vi "Clear message loop data.vi"(8 "error in (no error)":errorcluster, 11 "WAMP Client in":refnum<class "WAMP Client.lvclass">) -> (0 "error out":errorcluster, 3 "WAMP Clientout":refnum<class "WAMP Client.lvclass">)   [LabVIEW 2020, in "wamplv.lvlib" / "WAMP Client.lvclass"]
uses:
  WAMP Client.lvclass
  WAMP Client.lvclass/WAMP Client.ctl
  40994654-522d-4563-af25-94940d777c61.vi
  0b795402-a15f-4e31-95f5-2584284148d9.vi
  89e3171d-1602-4a33-a612-a198901d9ad6.vi
  a81c471f-8b4b-4529-bc43-673d3f160381.vi
  eb7fa446-2140-4dae-9b01-4fc8c6eccd10.vi
  40199801-e6b2-4318-9092-4349dd282dd3.vi
  6c0fe5e2-9903-440e-930a-5a8fedeab614.vi
  Private/Requests/ICallRequest/ICallRequest.lvclass
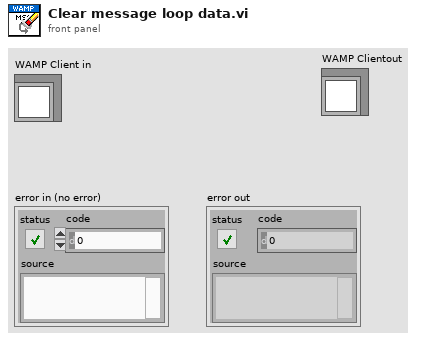
[diagram p1: front panel]
types:
  T1 = typedef "wamplv.lvlib/WAMP Client.lvclass/Message Loop Data.ctl" = cluster{"Last Request ID":u64, "Register Requests":map{u64, T2}, "Publish Requests":T3, "Endpoints Map":map{u64, T5}, "Call Requests":T6, "Subscription Requests":T7, "Subscriptions":T9, "Unsubscribe Requests":T11, "Random Request IDs":u64[], "Unregister requests map":T13}
  T2 = typedef "wamplv.lvlib/WAMP Client.lvclass/REGISTER Request Data.ctl" = cluster{"Procedure URI":string, "Options":string, "REGISTER result notifier":refnum<notifier>}
  T3 = typedef "wamplv.lvlib/WAMP Client.lvclass/Publish Requests Map.ctl" = map{u64, T4}
  T4 = typedef "wamplv.lvlib/WAMP Client.lvclass/PUBLISH Request Data.ctl" = cluster{"Topic URI":string, "Arguments":string, "ArgumentsKw":string, "Request Acknowledgement":bool, "Options":string, "Publish result notifier":refnum<notifier>}
  T5 = typedef "wamplv.lvlib/WAMP Client.lvclass/Endpoint Data.ctl" = cluster{"Procedure URI":string}
  T6 = typedef "wamplv.lvlib/WAMP Client.lvclass/CALL Request Map.ctl" = map{u64, refnum<class "ICallRequest.lvclass">}
  T7 = typedef "wamplv.lvlib/WAMP Client.lvclass/SUBSCRIBE Requests Map.ctl" = map{u64, T8}
  T8 = typedef "wamplv.lvlib/WAMP Client.lvclass/SUBSCRIBE Request Data.ctl" = cluster{"Topic":string, "Subscribe result notifer":refnum<notifier>, "Options":string}
  T9 = typedef "wamplv.lvlib/WAMP Client.lvclass/Subscriptions Map.ctl" = map{u64, T10}
  T10 = typedef "wamplv.lvlib/WAMP Client.lvclass/Subscription Details.ctl" = cluster{"Subscription ID":u64, "Topic":string, "Publication Received Event":refnum<user-event>, "Publication Received Notifier":refnum<notifier>, "Number of subscriptions":u64}
  T11 = typedef "wamplv.lvlib/WAMP Client.lvclass/Unsubscribe Requests Map.ctl" = map{u64, T12}
  T12 = typedef "wamplv.lvlib/WAMP Client.lvclass/UNSUBSCRIBE Request Data.ctl" = cluster{"Topic":string, "Unsubscrube result notifier":refnum<notifier>, "Options":string}
  T13 = typedef "wamplv.lvlib/WAMP Client.lvclass/Unregister requests map.ctl" = map{u64, T14}
  T14 = typedef "wamplv.lvlib/WAMP Client.lvclass/Unregister request.ctl" = cluster{"URI":string, "Unregister result notifier":refnum<notifier>, "Options":string}
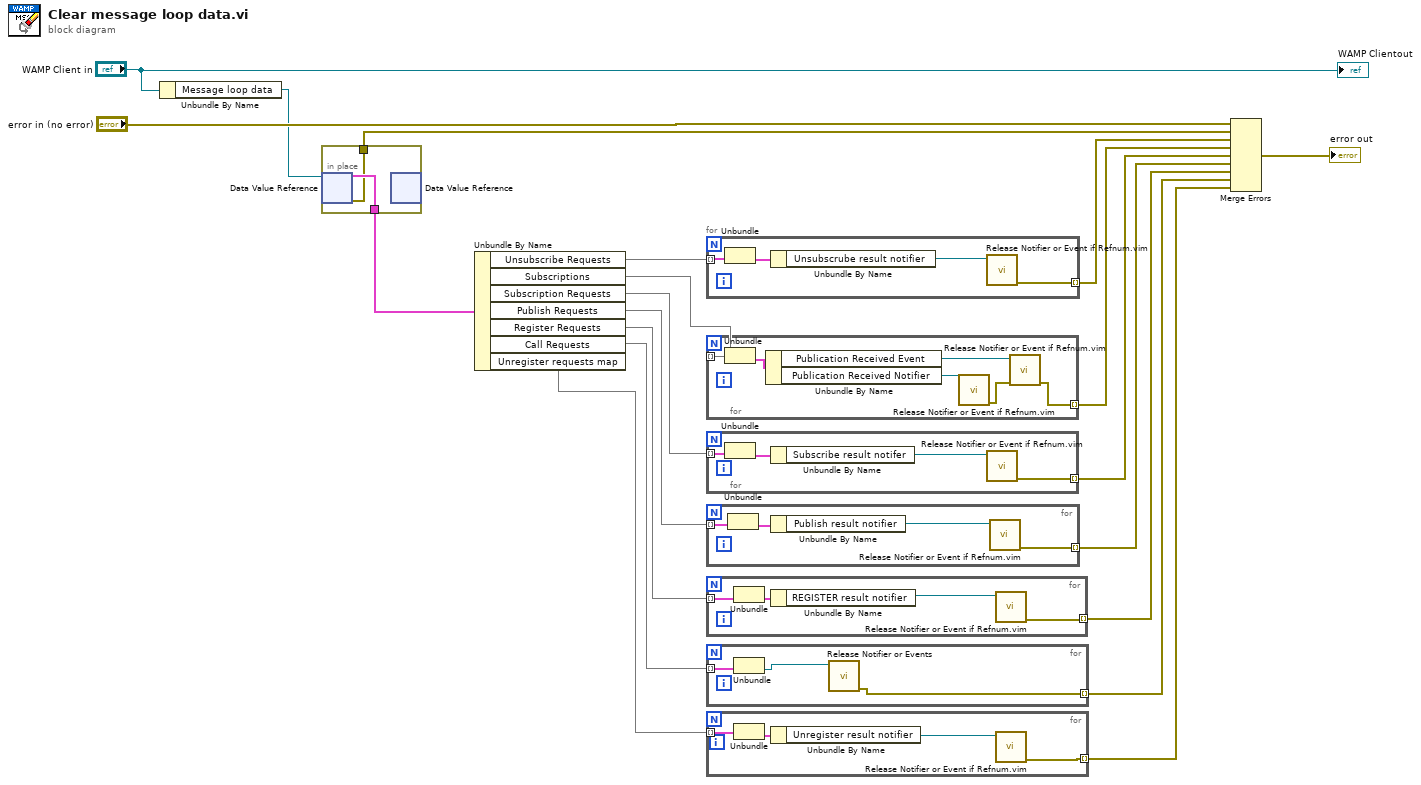
[diagram p0: block diagram]
diagram:
  n1 = Unbundle By Name("WAMP Client in") -> ("Message loop data"=w1:refnum<data-value>)
  n2 = in-place {
    in-place-border: [w22] -> w20
    in-place-border: [w21] -> w4
    n3 = in-place-dvr #1(w1) -> (w22:T1, w21:errorcluster)
    n4 = in-place-dvr #1() -> ()  [unwired: 1 in, 2 out]
  }
  n5 = Unbundle By Name(w20) -> ("Unsubscribe Requests"=w11:T11, "Subscriptions"=w10:T9, "Subscription Requests"=w9:T7, "Publish Requests"=w6:T3, "Register Requests"=w7:map{u64, T2}, "Call Requests"=w8:T6, "Unregister requests map"=w18:T13)
  n6 = for {
    tunnel: w11 -> [w26] mode=indexing
    tunnel: [w23] -> w12 mode=indexing
    n7 = Unbundle(w26) -> (w25:T12)  [unwired: 1 out]
    n8 = Unbundle By Name(w25) -> ("Unsubscrube result notifier"=w24:refnum<notifier>)
    n9 = call "Release Notifier or Event if Refnum.vim"("Notifier or Event in"=w24) -> ("error out"=w23:errorcluster)  [unwired: 10 in]
  }
  n10 = for {
    tunnel: w10 -> [w32] mode=indexing
    tunnel: [w30] -> w13 mode=indexing
    n11 = Unbundle(w32) -> (w31:T10)  [unwired: 1 out]
    n12 = Unbundle By Name(w31) -> ("Publication Received Event"=w29:refnum<user-event>, "Publication Received Notifier"=w28:refnum<notifier>)
    n13 = call "Release Notifier or Event if Refnum.vim"("Notifier or Event in"=w28) -> ("error out"=w27:errorcluster)  [unwired: 10 in]
    n14 = call "Release Notifier or Event if Refnum.vim"("error in (no error)"=w27, "Notifier or Event in"=w29) -> ("error out"=w30:errorcluster)  [unwired: 9 in]
  }
  n15 = for {
    tunnel: w9 -> [w36] mode=indexing
    tunnel: [w34] -> w14 mode=indexing
    n16 = Unbundle(w36) -> (w35:T8)  [unwired: 1 out]
    n17 = Unbundle By Name(w35) -> ("Subscribe result notifer"=w33:refnum<notifier>)
    n18 = call "Release Notifier or Event if Refnum.vim"("Notifier or Event in"=w33) -> ("error out"=w34:errorcluster)  [unwired: 10 in]
  }
  n19 = for {
    tunnel: w6 -> [w40] mode=indexing
    tunnel: [w38] -> w15 mode=indexing
    n20 = Unbundle(w40) -> (w39:T4)  [unwired: 1 out]
    n21 = Unbundle By Name(w39) -> ("Publish result notifier"=w37:refnum<notifier>)
    n22 = call "Release Notifier or Event if Refnum.vim"("Notifier or Event in"=w37) -> ("error out"=w38:errorcluster)  [unwired: 10 in]
  }
  n23 = for {
    tunnel: w7 -> [w44] mode=indexing
    tunnel: [w41] -> w16 mode=indexing
    n24 = Unbundle(w44) -> (w43:T2)  [unwired: 1 out]
    n25 = Unbundle By Name(w43) -> ("REGISTER result notifier"=w42:refnum<notifier>)
    n26 = call "Release Notifier or Event if Refnum.vim"("Notifier or Event in"=w42) -> ("error out"=w41:errorcluster)  [unwired: 10 in]
  }
  n27 = for {
    tunnel: w8 -> [w47] mode=indexing
    tunnel: [w45] -> w17 mode=indexing
    n28 = Unbundle(w47) -> ("CallRequest"=w46:refnum<class "ICallRequest.lvclass">)  [unwired: 1 out]
    n29 = call-dynamic "Release Notifier or Events.vi"("ICallRequest in"=w46) -> ("error out"=w45:errorcluster)  [unwired: 10 in]
  }
  n30 = for {
    tunnel: w18 -> [w51] mode=indexing
    tunnel: [w49] -> w19 mode=indexing
    n31 = Unbundle(w51) -> (w50:T14)  [unwired: 1 out]
    n32 = Unbundle By Name(w50) -> ("Unregister result notifier"=w48:refnum<notifier>)
    n33 = call "Release Notifier or Event if Refnum.vim"("Notifier or Event in"=w48) -> ("error out"=w49:errorcluster)  [unwired: 10 in]
  }
  n34 = Merge Errors("error in (no error)", w4, w12, w13, w14, w15, w16, w17, w19) -> (→"error out":errorcluster)
  "WAMP Clientout" <- "WAMP Client in"
